vi "Process Triggers.vi"(2 "acq":refnum<class "niVST Acquisition v1 FPGA.lvclass">=refnum) -> (10 "output valid":bool)   [LabVIEW 2023]
doc: "This VI reads the incoming start, advance, reference triggers, and configuration list step trigger (from software (if applicable), IO, or internally generated). Software triggers take precedence over other trigger types. the acquisition engine's \"ready for\" signals are also read. for example, \"ready for start\" is used to gate the input valid that is at the front of the DSP chain as well as to gate the start trigger sent to the acquisition engine.\n\nAfter the triggers are read, they are gated by the exported trigger events of the acquisition engine so that multiple triggers are not sent downstream while one is still in the pipeline since the acquisition engine can only process one trigger at a time. We discard triggers that are too closely spaced at this point.\n\nThe gated triggers that are sent to the acquisition engine are exported here alongside the \"ready for\" events.\n\n<b>output valid:</b> the start trigger marks the beginning of valid input data so we latch it here and use it as input valid of the DSP chain. it is cleared during DSP reset. this latched value is the output valid signal."
uses:
  <instrlib>/niVST/Reference FPGA/FPGA/Acquisition/v1/niVST Acquisition v1 FPGA.lvclass
  <instrlib>/niVST/Reference FPGA/FPGA/Shared/v1/niVST Shared v1 FPGA.lvclass
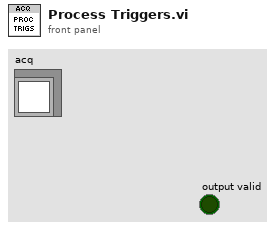
[diagram p1: front panel]
types:
  T1 = typedef "niVST Acquisition Alignment v1 FPGA.lvclass/Trigger Information.ctl" = cluster{"ready for start":bool, "ready for advance":bool, "ready for reference":bool, "start":bool, "start (direct)":bool, "advance":bool, "reference":bool, "reference (direct)":bool, "reference (async)":bool, "start trigger index":u16, "start trig delay (adc samples)":fxp<+,16,16>, "advance trigger index":u16, "adv trig delay (adc samples)":fxp<+,16,16>, "reference trigger index":u16, "ref trig delay (adc samples)":fxp<+,16,16>, "async ref trigger timestamp":T2, "iq data trigger timestamp":T2, "bypass addtl group delay?":u8, "ref trig is iq data trigger?":bool, "ref trig triggers immediately?":bool}
  T2 = typedef "niVST Shared Alignment v1 FPGA.lvclass/Time S128.64.ctl" = cluster{"msw":fxp<+/-,64,64>, "lsw":fxp<+,64,0>}
  T3 = typedef "niVST Sync Interface v1 FPGA.lvclass/Exported Trigger Information.ctl" = cluster{"use direct signal":bool, "direct signal":bool, "pre-conditioned signal":bool}
  T4 = typedef "niVST Acquisition Alignment v1 FPGA.lvclass/Trigger Adjustments.ctl" = cluster{"addtl sta trig delay (adc samples)":fxp<+/-,64,64>, "addtl adv trig delay (adc samples)":fxp<+/-,64,64>, "addtl ref trig delay (adc samples)":fxp<+/-,64,64>, "start trig offset (adc samples)":fxp<+/-,32,16>, "adv trig offset (adc samples)":fxp<+/-,32,16>, "ref trig offset (adc samples)":fxp<+/-,32,16>, "async ref timestamp offset (adc samples)":fxp<+/-,32,16>}
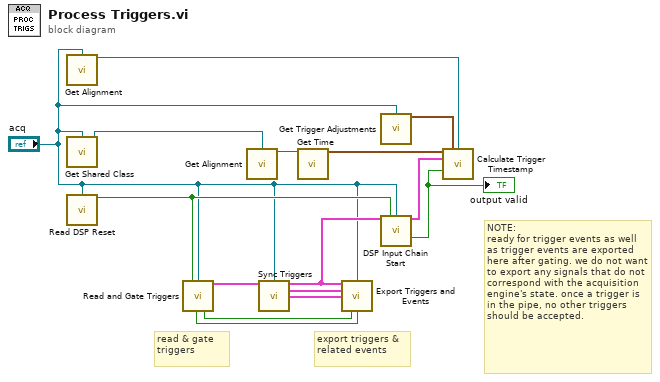
[diagram p0: block diagram]
diagram:
  # "read & gate triggers"
  # "export triggers & related events"
  # "NOTE:\nready for trigger events as well as trigger events are exported here after gating. we do not want to export any signals that do not correspond with the acquisition engine's state. once a trigger is in the pipe, no other triggers should be accepted."
  n1 = call-dynamic "Get Alignment.vi"("acq in"="acq") -> ("align"=w4:refnum<class "niVST Acquisition Alignment v1 FPGA.lvclass">)  [unwired: 14 in]
  n2 = call-dynamic "Get Shared Class.vi"("acq in"="acq") -> ("shared"=w3:refnum<class "niVST Shared v1 FPGA.lvclass">)  [unwired: 14 in]
  n3 = call-dynamic "Read DSP Reset.vi"("acq"="acq") -> ("dsp reset"=w11:bool)  [unwired: 14 in]
  n4 = call-dynamic "Read and Gate Triggers.vi"("reset"=w11, "acq"="acq") -> ("triggers"=w10:T1, "timer start trigger"=w5:bool, "clst"=w6:bool)  [unwired: 11 in]
  n5 = call-dynamic "Get Alignment.vi"("shared"=w3) -> ("align"=w15:refnum<class "niVST Shared Alignment v1 FPGA.lvclass">)  [unwired: 14 in]
  n6 = call-dynamic "Sync Triggers.vi"("triggers in"=w10, "acq"="acq") -> ("triggers out"=w9:T1, "sta trig info"=w8:T3, "ref trig info"=w7:T3)  [unwired: 11 in]
  n7 = call <instrlib>:"Get Time.vi"("align"=w15) -> ("time"=w13:T2)  [unwired: 14 in]
  n8 = call-dynamic "Export Triggers and Events.vi"("triggers"=w9, "acq"="acq", "sta trig info"=w8, "ref trig info"=w7, "clst"=w6, "timer start trigger"=w5) -> ()  [unwired: 10 in]
  n9 = call <instrlib>:"Get Trigger Adjustments.vi"("acq"="acq") -> ("trigger adjustments"=w2:T4)  [unwired: 14 in]
  n10 = call-dynamic "DSP Input Chain Start.vi"("triggers in"=w9, "reset"=w11, "acq"="acq") -> ("triggers out"=w12:T1, "output valid"=w14:bool)  [unwired: 11 in]
  "output valid" <- w14
  n11 = call <instrlib>:"Calculate Trigger Timestamp.vi"("time"=w13, "trigger adjustments"=w2, "acq align"=w4, "trigger info"=w12, "input valid"=w14) -> ()  [unwired: 11 in]
